vi "Floor 1 Temp FVG.vi"(7 "Mode":T1, 8 "Error In":errorcluster, 11 "Data In":dbl) -> (0 "Error Out":errorcluster, 3 "Data Out":dbl)   [LabVIEW 2014]
uses:
  Types/FVGFuncts.ctl
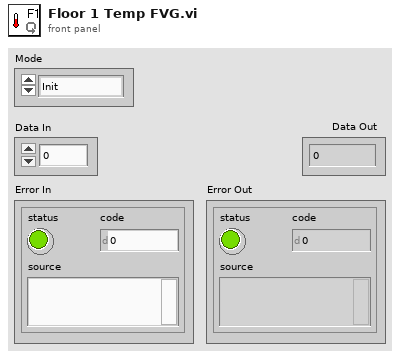
[diagram p1: front panel]
types:
  T1 = typedef "FVGFuncts.ctl" = enum16{"Init", "Set Data", "Get Data"}
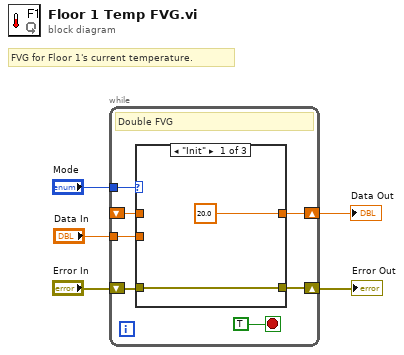
[diagram p0: block diagram]
diagram:
  # "FVG for Floor 1's current temperature."
  n1 = while {
    tunnel: "Mode" -> [w11]
    shift-right: [w9] -> w2
    shift-left: _ -> [w10]
    tunnel: "Data In" -> [w8]
    shift-right: [w6] -> w1
    shift-left: "Error In" -> [w7]
    stop <- TRUE stop-if-true
    # "Double FVG"
    n2 = case shown="\"Init\"" w11 {
      tunnel: w10 -> [_ _ w18]
      tunnel: [20.0 w16 w18] -> w9
      tunnel: w8 -> [_ w16 _]
      tunnel: w7 -> [w13 w15 w17]
      tunnel: [w13 w15 w17] -> w6
      frame "Init" {
      }
      frame "Set Data" {
      }
      frame "Get Data", Default {
      }
    }
  }
  "Data Out" <- w2
  "Error Out" <- w1
